vi "Adjust Phase for Frequency Change.vi"(0 "SV Signal in":refnum<class "SV Signal.lvclass">, 5 "time offset at state":dbl, 7 "previous signal state":variant, 11 "error in (no error)":errorcluster, 12 "signal state in":variant) -> (4 "SV Signal out":refnum<class "SV Signal.lvclass">, 14 "signal state out":variant, 15 "error out":errorcluster)   [LabVIEW 2017, in "SV Signal.lvclass"]
uses:
  <vilib>/addons/_NISVFA/_Generation/Signal Generation/SV Signal/SV Signal.lvclass
  <vilib>/addons/_NISVFA/_Generation/Signal Generation/SV Signal/SV Signal.lvclass/SV Signal.ctl
  <vilib>/addons/_NISVFA/_Generation/Signal Generation/SV Signal/sv_Signal State Attribute.ctl
  <vilib>/addons/_NISVFA/_Generation/SoundVib_Generation.lvlib
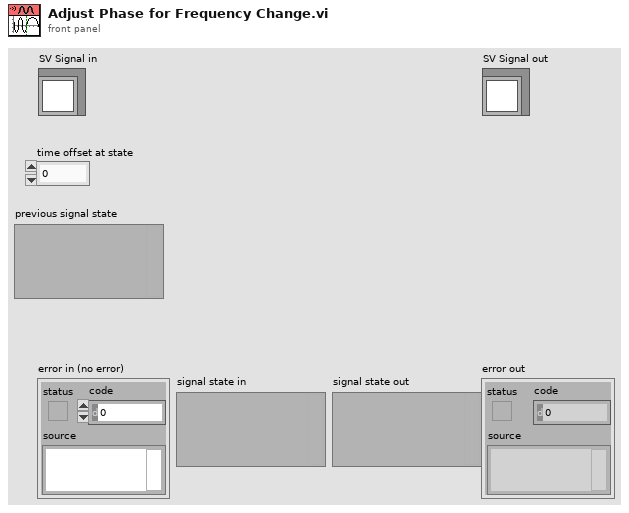
[diagram p1: front panel]
types:
  T1 = typedef "SV Signal.lvclass/sv_Signal State Attribute.ctl" = string
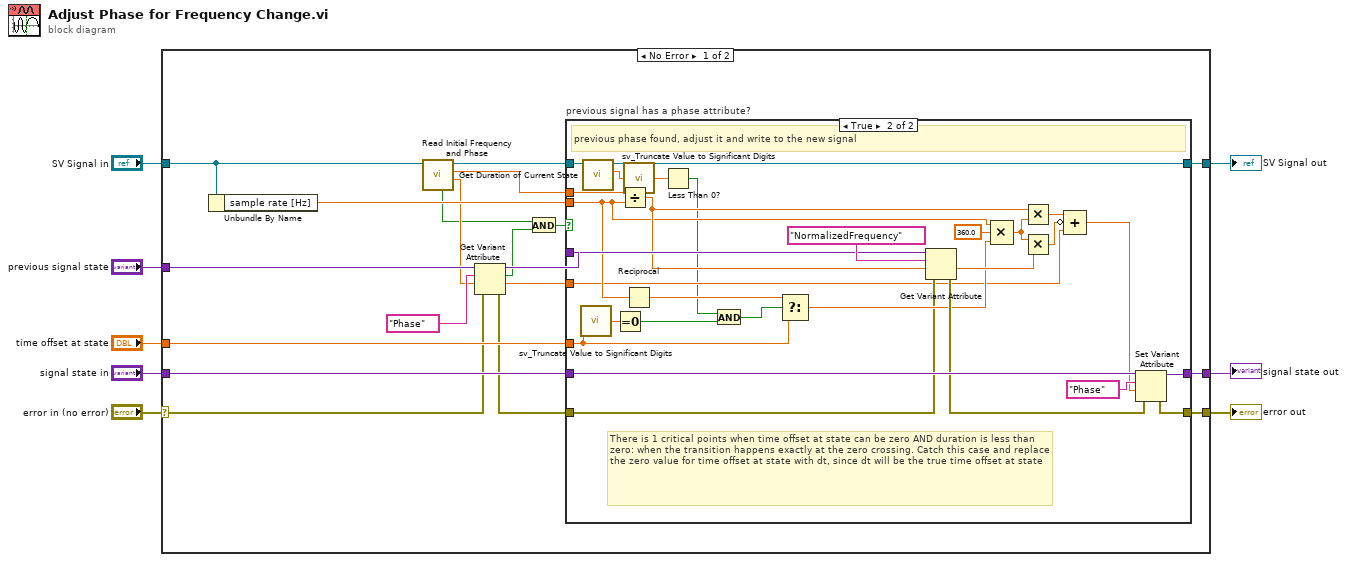
[diagram p0: block diagram]
diagram:
  n1 = case shown="No Error" "error in (no error)" {
    selector: "error in (no error)" -> [w21 w62]
    tunnel: [w27 w62] -> w7
    tunnel: [w25 w61] -> w5
    tunnel: "SV Signal in" -> [w20 w61]
    tunnel: [w26 w60] -> w4
    tunnel: "signal state in" -> [w22 w60]
    tunnel: "previous signal state" -> [w23 _]
    tunnel: "time offset at state" -> [w24 _]
    frame No Error {
      n2 = Unbundle By Name(w20) -> ("sample rate [Hz]"=w19:dbl)
      n3 = call-dynamic "Read Initial Frequency and Phase.vi"("SV Signal in"=w20) -> ("initial phase"=w12:dbl, "initial frequency"=w13:dbl, "SV Signal out"=w14:refnum<class "SV Signal.lvclass">, "found?"=w10:bool)  [unwired: 6 in, 1 out]
      n4 = Get Variant Attribute(Variant=w23, name=T1 "Phase" ("attribute"), default value (empty Variant)=w12, error in=w21) -> (duplicate Variant=w17:variant, found=w11:bool, value=w15:dbl, error out=w16:errorcluster)
      n5 = And(x=w10, y=w11) -> (x .and. y?=w9:bool)
      n6 = case "previous signal has a phase attribute?" shown="True" w9 {
        tunnel: w17 -> [_ w58]
        tunnel: w13 -> [_ w57]
        tunnel: w19 -> [_ w44]
        tunnel: w16 -> [w28 w37]
        tunnel: [w28 w47] -> w27
        tunnel: [w30 w34] -> w25
        tunnel: w14 -> [w30 w35]
        tunnel: [w29 w49] -> w26
        tunnel: w22 -> [w29 w50]
        tunnel: w15 -> [_ w36]
        tunnel: w24 -> [_ w39]
        frame False {
          # "no previous phase attribute, don't adjust phase"
        }
        frame True {
          # "There is 1 critical points when time offset at state can be zero AND duration is less than zero: when the transition happens exactly at the zero crossing. Catch this case and replace the zero value for time offset at state with dt, since dt will be the true time offset at state"
          # "previous phase found, adjust it and write to the new signal"
          n7 = call <vilib>:"sv_Truncate Value to Significant Digits.vi"("value"=w39) -> ("truncated value"=w38:dbl)  [unwired: 14 in]
          n8 = call-dynamic "Get Duration of Current State.vi"("signal configuration"=w35) -> ("current state duration [s]"=w32:dbl, "signal configuration"=w34:refnum<class "SV Signal.lvclass">)  [unwired: 9 in]
          n9 = Equal To 0?(x=w38) -> (x = 0?=w41:bool)
          n10 = Divide(x=w57, y=w44) -> (x/y=w56:dbl)
          n11 = call <vilib>:"sv_Truncate Value to Significant Digits.vi"("value"=w32) -> ("truncated value"=w31:dbl)  [unwired: 14 in]
          n12 = Reciprocal(x=w44) -> (1/x=w43:dbl)
          n13 = Less Than 0?(x=w31) -> (x < 0?=w33:bool)
          n14 = And(x=w33, y=w41) -> (x .and. y?=w40:bool)
          n15 = Select(t=w43, s=w40, f=w39) -> (s? t:f=w42:dbl)
          n16 = Get Variant Attribute(Variant=w58, name=T1 "NormalizedFrequency" ("attribute"), default value (empty Variant)=w56, error in=w37) -> (value=w55:dbl, error out=w48:errorcluster)  [unwired: 2 out]
          n17 = Compound Arithmetic op=MULTIPLY(w44, 360.0 ("x"), w42) -> (w54:dbl)
          n18 = Multiply(x=w56, y=w54) -> (x*y=w53:dbl)
          n19 = Multiply(x=w54, y=w55) -> (x*y=w52:dbl)
          n20 = Compound Arithmetic op=ADD(w53, invert w52, w36) -> (w45:dbl)
          n21 = Set Variant Attribute(Variant=w50, name=T1 "Phase" ("attribute"), value=w45, error in=w48) -> (Variant out=w49:variant, error out=w47:errorcluster)  [unwired: 1 out]
        }
      }
    }
    frame Error {
    }
  }
  "error out" <- w7
  "SV Signal out" <- w5
  "signal state out" <- w4
